vi "FindPeakFreq.vi"(5 "magnitude":cluster{"f0":dbl, "df":dbl, "magnitude":dbl[]} {"magnitude" format="%.2p"; "f0" format="%0.2p"; "df" format="%0.2p"}) -> (1 "Max":dbl, 2 "output cluster":cluster{"f0":dbl, "df":dbl, "magnitude":dbl[]})   [LabVIEW 2020]
panel:
  out "reversed array":dbl[](array[numeric])
  out "Waveform Graph":cluster{"f0":dbl, "df":dbl, "magnitude":dbl[]}(graph)
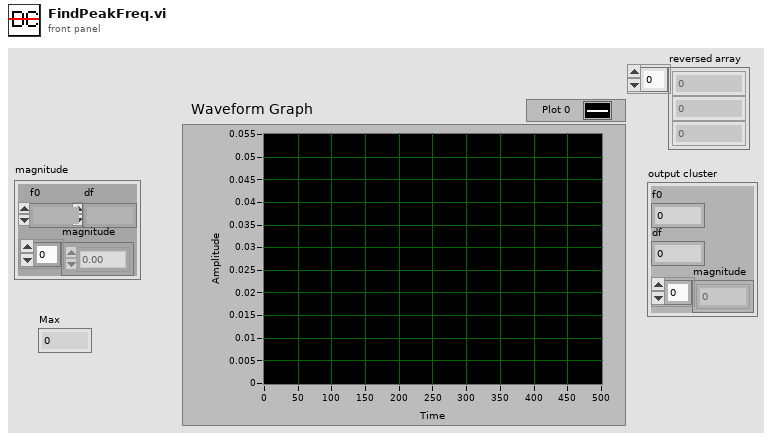
[diagram p1: front panel]
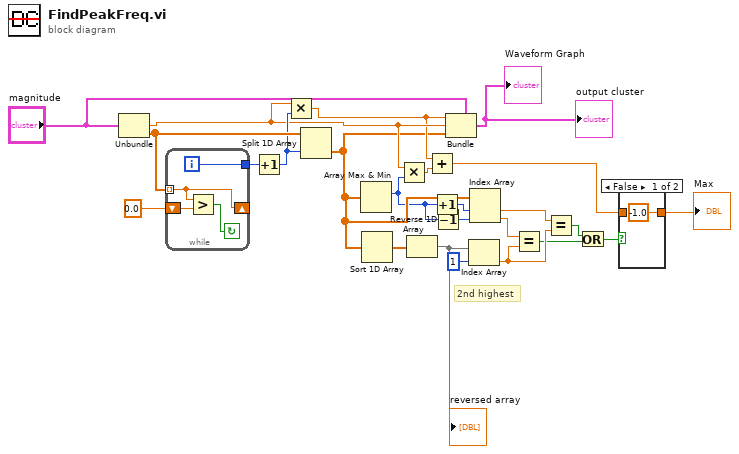
[diagram p0: block diagram]
diagram:
  # "2nd highest"
  n1 = Unbundle("magnitude") -> ("df"=w18:dbl, "magnitude"=w23:dbl[])  [unwired: 1 out]
  n2 = while {
    tunnel: w23 -> [w27] mode=indexing
    shift-right: [w27] -> _
    shift-left: 0.0 -> [w28]
    tunnel: [w25] -> w20
    i -> [w25]
    stop <- w26 continue-if-true
    n3 = Greater?(x=w27, y=w28) -> (0:w26:bool)
  }
  n4 = Increment(x=w20) -> (x+1=w19:i32)
  n5 = Multiply(x=w18, y=w19) -> (x*y=w16:dbl)
  n6 = Split 1D Array(array=w23, index=w19) -> (second subarray=w12:dbl[])  [unwired: 1 out]
  n7 = Array Max & Min(array=w12) -> (max index (indices)=w9:i32)  [unwired: 3 out]
  n8 = Sort 1D Array(array=w12) -> (sorted array=w15:dbl[])
  n9 = Multiply(x=w18, y=w9) -> (x*y=w17:dbl)
  n10 = Reverse 1D Array(array=w15) -> (reversed array=w14:dbl[])
  "reversed array" <- w14
  n11 = Add(x=w16, y=w17) -> (x+y=w2:dbl)
  n12 = Increment(x=w9) -> (x+1=w11:i32)
  n13 = Decrement(x=w9) -> (x-1=w10:i32)
  n14 = Bundle(cluster="magnitude", "f0"=w16, "df"=w18, "magnitude"=w12) -> (→"Waveform Graph" →"output cluster":cluster{"f0":dbl, "df":dbl, "magnitude":dbl[]})
  n15 = Index Array(array=w14, index=1) -> (element=w7:dbl)
  n16 = Index Array(array=w12, index #1=w11, index #2=w10) -> (element #1=w6:dbl, element #2=w8:dbl)
  n17 = Equal?(x=w8, y=w7) -> (x = y?=w4:bool)
  n18 = Equal?(x=w6, y=w7) -> (x = y?=w5:bool)
  n19 = Or(x=w5, y=w4) -> (x .or. y?=w3:bool)
  n20 = case shown="False" w3 {
    tunnel: w2 -> [_ w30]
    tunnel: [-1.0 w30] -> w1
    frame False {
    }
    frame True {
    }
  }
  "Max" <- w1
